vi "HEWH Su0 Heating Event and Draw Same Time.vi"(8 "error in (no error)":errorcluster, 10 "Draw Index in":i32[](array[numeric]), 11 "Heating Index in":i32[][](array[numeric])) -> (0 "error out":errorcluster, 2 "SUo Start Index":i32)   [LabVIEW 2023]
panel:
  out "DrawCausedHeat":u8
  in  "Water Heater Type":string(combo)
  in  "Draw Index (30 Gal Std Electric)":i32[](array[numeric])=[2841, 3165]
  in  "Heating Index (30 Gal Std Electric)":i32[][](array[numeric])=[[221, 1180], [2992, 3498], [13926, 14456], [16493, 16662], [17883, 17999], [22467, 22635], [24007, 24372]]
  in  "Draw Index (50 Gal Std Electric)":i32[](array[numeric])=[3093, 3417]
  in  "Heating Index (50 Gal Std Electric)":i32[][](array[numeric])=[[338, 744], [755, 2075], [14195, 15239], [23885, 25361]]
  in  "Draw Index (Gas Storage)":i32[](array[numeric])=[3121, 3449]
  in  "Gas Heating Index (Gas Storage)":i32[][](array[numeric])=[[47, 1107], [1242, 1362], [1732, 1779], [3170, 3610], [14187, 14722], [15804, 16042], [16746, 16789], [17898, 18000], [18197, 18237], [22250, 22347], [22837, 22939], [23404, 23491], [23961, 24047], [24507, 25023]]
  in  "Heat Pump (Heat Pump)":i32[](array[numeric])=[2845, 3169]
  in  "Heat Pump (Heat Pump)":i32[][](array[numeric])=[[500, 4543], [14227, 17075], [24131, 26311]]
  # "Debug Data"
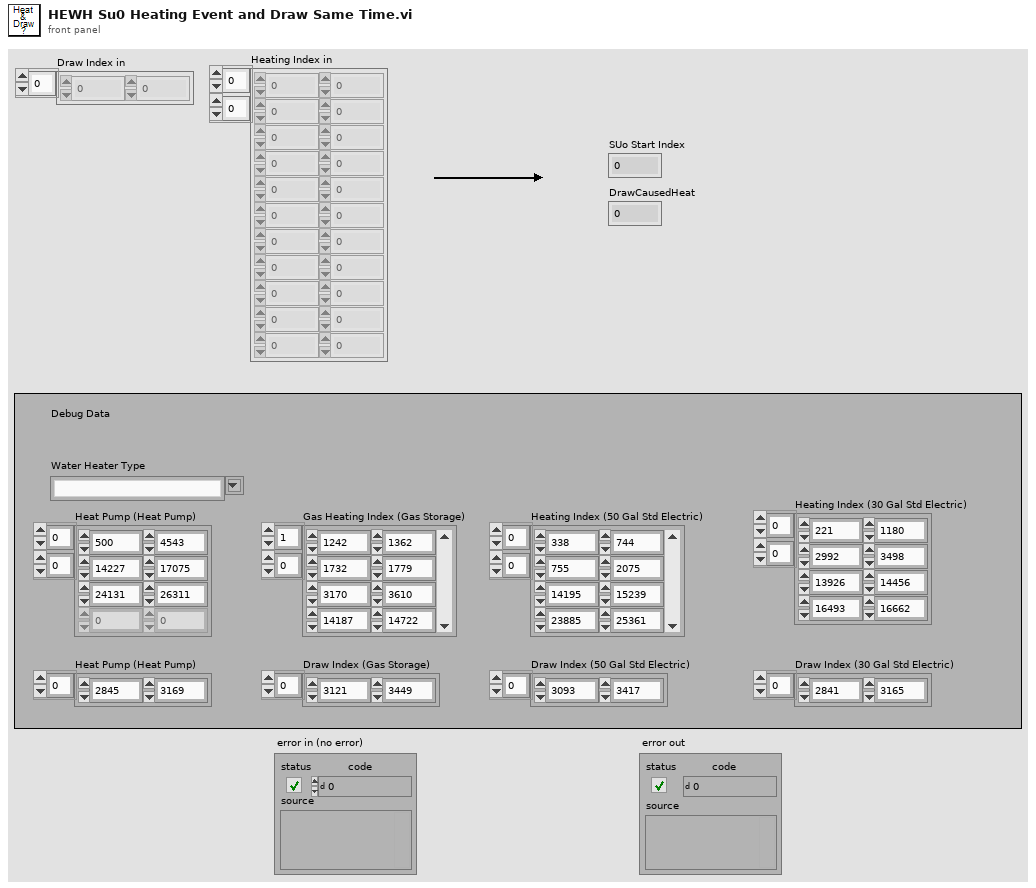
[diagram p1: front panel]
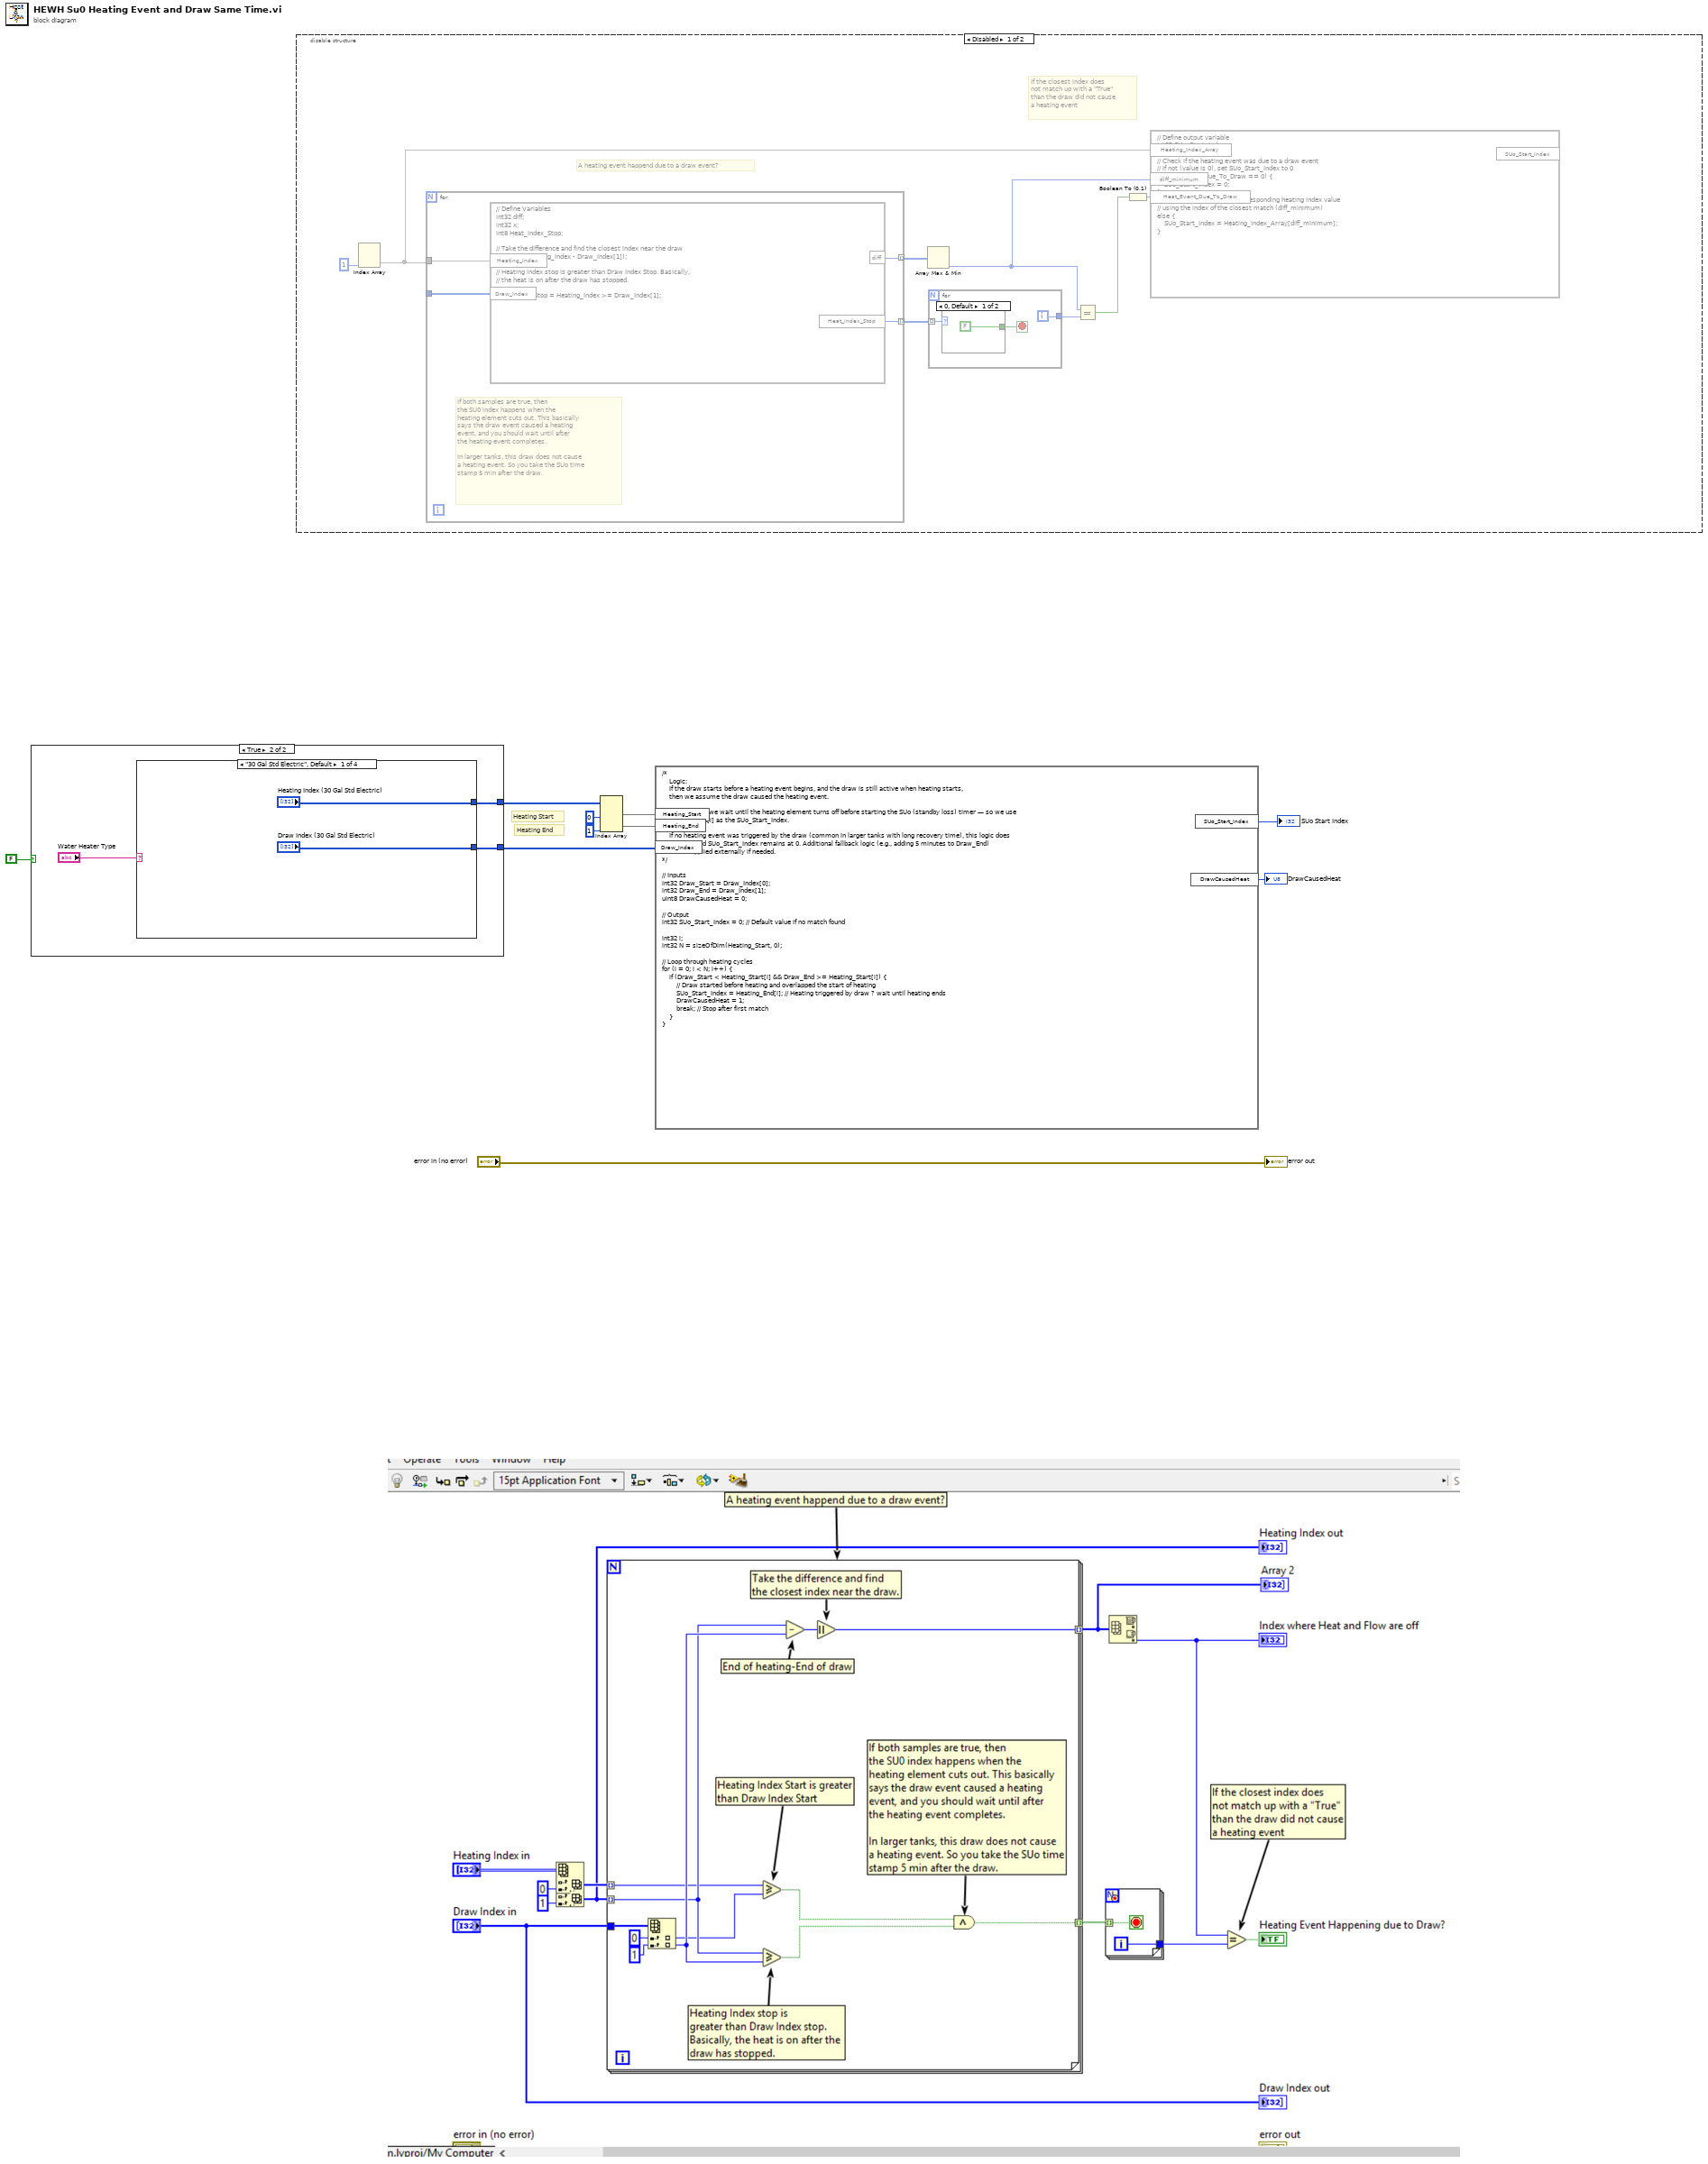
[diagram p0: block diagram]
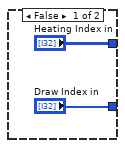
[diagram p2: hidden frame]
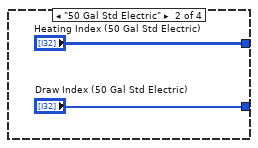
[diagram p3: hidden frame]
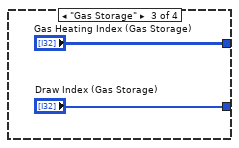
[diagram p4: hidden frame]
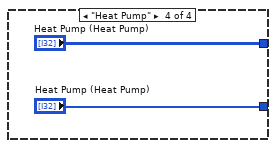
[diagram p5: hidden frame]
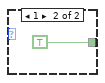
[diagram p6: hidden frame]
diagram:
  # "Heating End"
  # "Heating Start"
  n1 = case shown="True" FALSE {
    tunnel: ["Heating Index in" w14] -> w4
    tunnel: ["Draw Index in" w13] -> w3
    frame False {
    }
    frame True {
      n2 = case shown="\"30 Gal Std Electric\", Default" "Water Heater Type" {
        tunnel: ["Heating Index (30 Gal Std Electric)" "Heating Index (50 Gal Std Electric)" "Gas Heating Index (Gas Storage)" "Heat Pump (Heat Pump)"] -> w14
        tunnel: ["Draw Index (30 Gal Std Electric)" "Draw Index (50 Gal Std Electric)" "Draw Index (Gas Storage)" "Heat Pump (Heat Pump)"] -> w13
        frame "30 Gal Std Electric", Default {
        }
        frame "50 Gal Std Electric" {
        }
        frame "Gas Storage" {
        }
        frame "Heat Pump" {
        }
      }
    }
  }
  n3 = disable-structure shown="Disabled" {
    frame Disabled {
      # "If the closest index does\nnot match up with a \"True\"\nthan the draw did not cause\na heating event"
      # "A heating event happend due to a draw event?"
      n4 = Index Array "Index Array"(index (col)=1) -> (element=w28)  [unwired: 2 in]
      n5 = for {
        tunnel: _ -> [w38]
        tunnel: w28 -> [w40]
        tunnel: [w39] -> w30 mode=indexing
        tunnel: [w37] -> w24 mode=indexing
        # "If both samples are true, then\nthe SU0 index happens when the\nheating element cuts out. This basically\nsays the draw event caused a heating\nevent, and you should wait until after\nthe heating event completes.\n\nIn larger tanks, this draw does not cause\na heating event. So you take the SUo time\nstamp 5 min after the draw."
        n6 = formula code="// Define Variables\nint32 diff;\nint32 x;\nint8 Heat_Index_Stop;\n\n// Take the difference and find the closest index near the draw\ndiff = abs(Heating_Index - Draw_Index[1]);\n\n// Heating Index stop is greater than Draw Index Stop. Basically,\n// the heat is on after the draw has stopped.\n\nHeat_Index_Stop = Heating_Index >= Draw_Index[1];"("Heating_Index"=w40, "Draw_Index"=w38) -> ("diff"=w39:i32, "Heat_Index_Stop"=w37:i8)
      }
      n7 = Array Max & Min(array=w30) -> (min index (indices)=w27:i32)  [unwired: 3 out]
      n8 = for {
        tunnel: w24 -> [w33] mode=indexing
        tunnel: [w34] -> w31
        i -> [w34]
        stop <- w32 stop-if-true
        n9 = case shown="0, Default" w33 {
          tunnel: [FALSE TRUE] -> w32
          frame 0, Default {
          }
          frame 1 {
          }
        }
      }
      n10 = Equal?(x=w27, y=w31) -> (x = y?=w26:bool)
      n11 = Boolean To (0,1)(Boolean=w26) -> (0, 1=w25:i16)
      n12 = formula code="// Define output variable\nint32 SUo_Start_Index;\n\n// Check if the heating event was due to a draw event\n// If not (value is 0), set SUo_Start_Index to 0\nif (Heat_Event_Due_To_Draw == 0) {\n    SUo_Start_Index = 0;\n} \n// Otherwise, set it to the corresponding heating index value \n// using the index of the closest match (diff_minimum)\nelse {\n    SUo_Start_Index = Heating_Index_Array[diff_minimum];\n}"("Heating_Index_Array"=w28, "diff_minimum"=w27, "Heat_Event_Due_To_Draw"=w25) -> ()  [unwired: 1 out]
    }
    frame Enabled {
    }
  }
  n13 = Index Array "Index Array"(array=w4, index (col) #1=0 ("disabled index (col)"), index (col) #2=1 ("index (col)")) -> (element #1=w7:i32[], element #2=w6:i32[])  [unwired: 2 in]
  n14 = formula code="/*\n    Logic:\n    If the draw starts before a heating event begins, and the draw is still active when heating starts,\n    then we assume the draw caused the heating event.\n\n    In that case, we wait until the heating element turns off before starting the SUo (standby loss) timer — so we use\n    Heating_End[i] as the SUo_Start_Index.\n\n    If no heating event was triggered by the draw (common in larger tanks with long recovery time), this logic does\n    nothing, and SUo_Start_Index remains at 0. Additional fallback logic (e.g., adding 5 minutes to Draw_End)\n    can be applied externally if needed.\n*/\n\n// Inputs\nint32 Draw_Start = Draw_Index[0];\nint32 Draw_End = Draw_Index[1];\nuInt8 DrawCausedHeat = 0;\n\n// Output\nint32 SUo_Start_Index = 0; // Default value if no match found\n\nint32 i;\nint32 N = sizeOfDim(Heating_Start, 0);\n\n// Loop through heating cycles\nfor (i = 0; i < N; i++) {\n    if (Draw_Start < Heating_Start[i] && Draw_End >= Heating_Start[i]) {\n        // Draw started before heating and overlapped the start of heating\n        SUo_Start_Index = Heating_End[i]; // Heating triggered by draw ? wait until heating ends\n        DrawCausedHeat = 1;\n        break; // Stop after first match\n    }\n}"("Heating_Start"=w7, "Draw_Index"=w3, "Heating_End"=w6) -> ("SUo_Start_Index"=→"SUo Start Index":i32, "DrawCausedHeat"=→"DrawCausedHeat":u8)
  "error out" <- "error in (no error)"
